vi "Power.vi"   [LabVIEW 2013, in "NI_EP_Basic.lvlib"]
doc: "Calculates the power values from a voltage and current signal. Wire data to the <B>voltage waveform</B> input or the <B>current waveform</B> input to determine the polymorphic instance to use or manually select the instance."
uses:
  <vilib>/addons/Electrical Power/Basic/NI_EP_Basic.lvlib
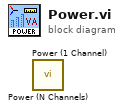
[diagram p0: block diagram]
diagram:
  n1 = call <vilib>:"Power (N Channels).vi"() -> ()  [unwired: 10 in, 2 out]
  n2 = call <vilib>:"Power (1 Channel).vi"() -> ()  [unwired: 10 in, 2 out]
